vi "Idle Connection - Server.vi"(0 "listener ID":refnum<k5>, 1 "connection ID":refnum<k5>, 2 "Message to Send":string="Starting Tests....", 3 "error in (no error)":errorcluster) -> (7 "data out":string, 10 "error out":errorcluster)   [LabVIEW 2020]
doc: "Tests ports in direction of cliend to server"
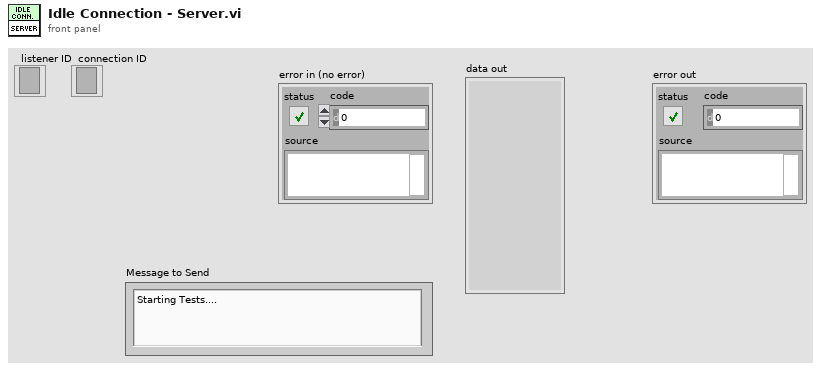
[diagram p1: front panel]
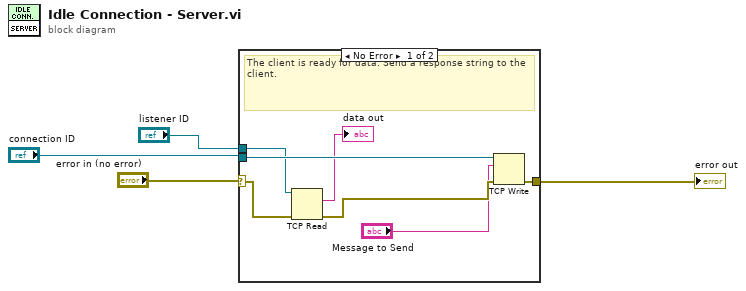
[diagram p0: block diagram]
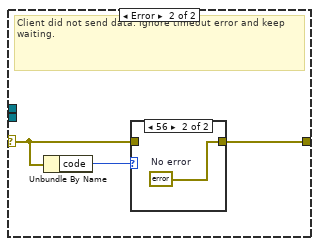
[diagram p2: hidden frame]
diagram:
  n1 = case shown="No Error" "error in (no error)" {
    selector: "error in (no error)" -> [w8 w14]
    tunnel: [w9 w12] -> w4
    tunnel: "connection ID" -> [w11 _]
    tunnel: "listener ID" -> [w10 _]
    frame No Error {
      # "The client is ready for data. Send a response string to the client."
      n2 = TCP Read(connection ID=w10, error in (no error)=w8) -> (data out=→"data out":string, error out=w7:errorcluster)  [unwired: 3 in, 1 out]
      n3 = TCP Write(connection ID=w11, data in="Message to Send", error in (no error)=w7) -> (error out=w9:errorcluster)  [unwired: 1 in, 2 out]
    }
    frame Error {
      # "Client did not send data. Ignore timeout error and keep waiting."
      n4 = Unbundle By Name(w14) -> ("code"=w13:i32)
      n5 = case shown="56" w13 {
        tunnel: w14 -> [w15 _]
        tunnel: [w15 w16] -> w12
        frame Default {
        }
        frame 56 {
          w16 = errorcluster {"status"=FALSE, "code"=0, "source"=""}  # No error
        }
      }
    }
  }
  "error out" <- w4
